vi "Global 1.vi"() -> ()   [LabVIEW 2022 SP3]
panel:
  out "ALS":bool
  out "Seq State":string
  in  "Log Period":dbl=900.0
  out "Signal names":string[][](array[string])
  in  "RT IP":string="localhost"
  out "Hw file":string
  out "Exit":bool
  out "CDAQ":bool
  out "RT Connect":bool
  out "writer name":refnum<k21>
  out "Restart Log":bool
  out "Datalog":string
  out "Log":bool
  out "Start DAQ":bool
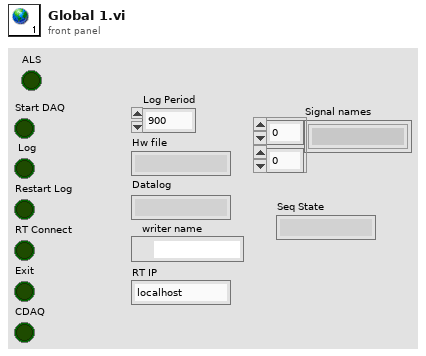
[diagram p1: front panel]
diagram:
